vi "Get Port Properties.vi"(8 "error in":errorcluster, 11 "custom device ref":T2 format="%.0x") -> (0 "error out":errorcluster, 2 "port properties out":T1, 3 "custom device ref out":T2 format="%.0x")   [LabVIEW 2020, in "AIM ARINC 664 Scripting.lvlib"]
uses:
  AIM ARINC 664 Scripting.lvlib
  <vilib>/NI VeriStand/Custom Device API/Custom Device Item Ref.ctl
  Import/_typedefs/port_setup.ctl
  Import/AIM ARINC 664 Import.lvlib
  <vilib>/NI VeriStand/Custom Device API/Custom Device API.lvlib
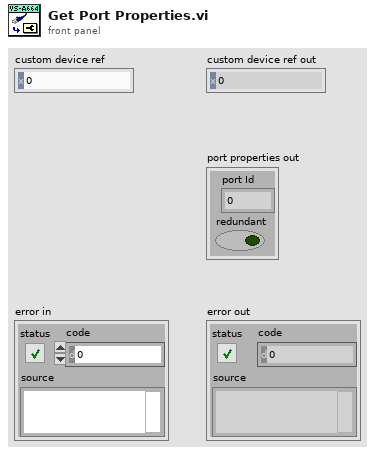
[diagram p1: front panel]
types:
  T1 = typedef "AIM ARINC 664 Import.lvlib/port_setup.ctl" = cluster{"port Id":u32, "redundant":bool}
  T2 = typedef "Custom Device API.lvlib/Custom Device Item Ref.ctl" = u64
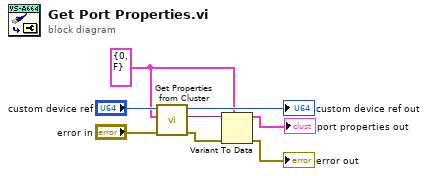
[diagram p0: block diagram]
diagram:
  w3 = T1 {"port Id"=0, "redundant"=FALSE} ("portSetup")
  n1 = call "Get Properties from Cluster.vi"("error in"="error in", "Variant Cluster"=w3, "custom device ref in"="custom device ref") -> ("error out"=w4:errorcluster, "data"=w5:variant, "custom device ref out"=→"custom device ref out":T2)  [unwired: 5 in, 1 out]
  n2 = Variant To Data(error in=w4, type=w3, Variant=w5) -> (data=→"port properties out":T1, error out=→"error out":errorcluster)
